vi "SubVI_WaitNthLoops.vi"(2 "error in (no error)":errorcluster, 3 "Wait":bool=TRUE, 4 "loop execution\n(milliseconds)":i32=20, 5 "milliseconds to wait":i32=12) -> (0 "error out":errorcluster, 1 "Continue":bool)   [LabVIEW 2017]
doc: "Input a true to start the waiter\n\nContinue indicates if you can continue with your code (if it is false, you are still waiting)"
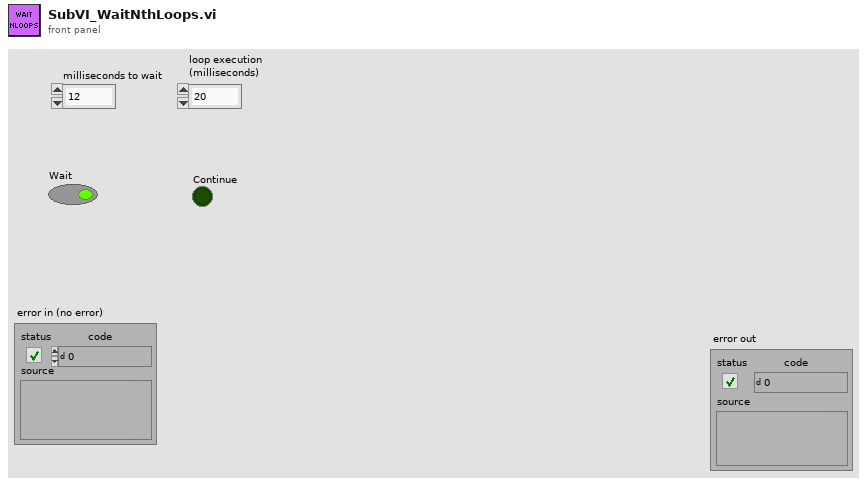
[diagram p1: front panel]
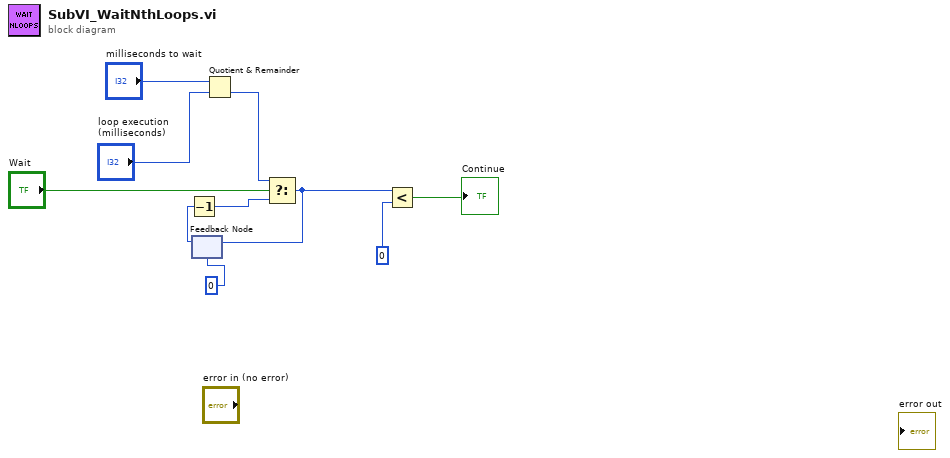
[diagram p0: block diagram]
diagram:
  n1 = feedback #1(0 ("Number of loops to wait \nbetween each change.")) -> (w10:i32)
  n2 = Decrement(x=w10) -> (x-1=w8:i32)
  n3 = Quotient & Remainder(x="milliseconds to wait", y="loop execution\n(milliseconds)") -> (floor(x/y)=w5:i32)  [unwired: 1 out]
  n4 = Select(t=w5, s="Wait", f=w8) -> (s? t:f=w3:i32)
  n5 = feedback-in #1(w3) -> ()
  n6 = Less?(x=w3, y=0) -> (x < y?=→"Continue":bool)
